vi "dvp Vi Set Strobe Delay.vi"(10 "StrobeDelay":dbl, 11 "handle":u32) -> (3 "function return":u32(ring))   [LabVIEW 2018, in "LabViewDVPCamera.lvlib"]
doc: "LabviewDvp2Api dvpStatus dvpViSetStrobeDelay(dvpHandle handle, double StrobeDelay);"
uses:
  LabViewDVPCamera.lvlib
  LabViewDVPCamera/LabViewDVPCamera.dll
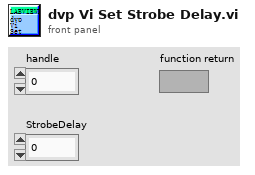
[diagram p1: front panel]
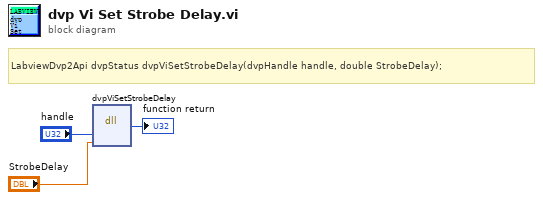
[diagram p0: block diagram]
diagram:
  # "LabviewDvp2Api dvpStatus dvpViSetStrobeDelay(dvpHandle handle, double StrobeDelay);"
  n1 = dll-call lib="C:/Program Files (x86)/DVP2 Labview cn 64/Sample/LabViewDVPCamera/LabViewDVPCamera.*" fn="dvpViSetStrobeDelay"("handle"="handle", "StrobeDelay"="StrobeDelay") -> (→"function return":u32)  [unwired: 5 in, 2 out]
